vi "PNA_Configure Marker.vi"(0 "VISA resource name":refnum<visa-resource-name>, 1 "Channel (1)":i32=1, 2 "Trace (1)":i32=1, 3 "Marker (1)":i32=1, 5 "Marker State (F: Disabled)":bool, 9 "Mkr Freq":dbl format="%^.2e", 11 "error in (no error)":errorcluster, 13 "Units(Hz)":u32(ring) items=["Hz"=1, "MHz"=1000000, "GHz"=1000000000]) -> (4 "VISA resource name out":refnum<visa-resource-name>, 15 "error out":errorcluster)   [LabVIEW 2018, in "Agilent ENA Series.lvlib"]
doc: "Configures marker."
uses:
  Agilent ENA Series.lvlib
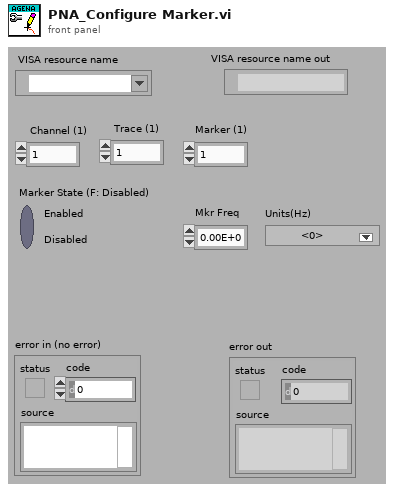
[diagram p1: front panel]
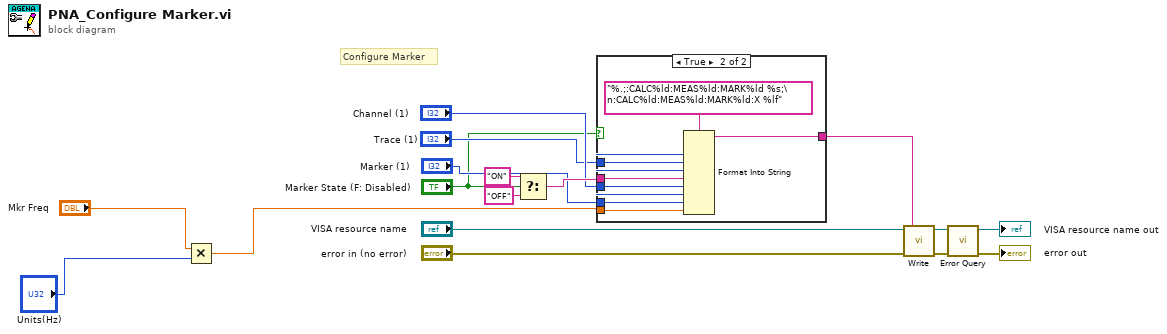
[diagram p0: block diagram]
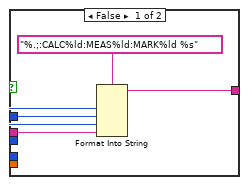
[diagram p2: hidden frame]
diagram:
  # "Configure Marker"
  n1 = Multiply(x="Mkr Freq", y="Units(Hz)") -> (x*y=w1:dbl)
  n2 = Select(t="ON", s="Marker State (F: Disabled)", f="OFF") -> (s? t:f=w13:string)
  n3 = case shown="True" "Marker State (F: Disabled)" {
    tunnel: w13 -> [w23 w30]
    tunnel: w1 -> [_ w29]
    tunnel: "Channel (1)" -> [w22 w28]
    tunnel: "Marker (1)" -> [w21 w27]
    tunnel: "Trace (1)" -> [w20 w26]
    tunnel: [w18 w24] -> w5
    frame False {
      n4 = Format Into String(format string="%.;:CALC%ld:MEAS%ld:MARK%ld %s", w22, w20, w21, w23) -> (resulting string=w18:string)  [unwired: 2 in, 1 out]
    }
    frame True {
      n5 = Format Into String(format string="%.;:CALC%ld:MEAS%ld:MARK%ld %s;\n:CALC%ld:MEAS%ld:MARK%ld:X %lf", w28, w26, w27, w30, w28, w26, w27, w29) -> (resulting string=w24:string)  [unwired: 2 in, 1 out]
    }
  }
  n6 = call "Write.vi"("error in (no error)"="error in (no error)", "String ()"=w5, "VISA resource name"="VISA resource name") -> ("error out"=w9:errorcluster, "VISA resource name out"=w10:refnum<visa-resource-name>)  [unwired: 6 in, 1 out]
  n7 = call "Error Query.vi"("error in (no error)"=w9, "VISA resource name"=w10) -> ("error out"=→"error out":errorcluster, "VISA resource name out"=→"VISA resource name out":refnum<visa-resource-name>)  [unwired: 6 in, 2 out]
